vi "Parameter_2nd_part.vi"(6 "Biometry Configuration":T1, 7 "测试？":bool, 8 "Error In":errorcluster caption="错误输入", 9 "A\\B":dbl[](array[numeric]), 10 "Correction Data 2nd":dbl[](array[numeric]), 11 "S":dbl[](array[numeric])) -> (0 "Error Out":errorcluster caption="错误输出", 1 "最值位置":dbl, 2 "开始位置":dbl, 3 "视网膜厚度":dbl)   [LabVIEW 2015, in "Boimetry Processing.lvlib"]
doc: "计算眼后节结果。"
uses:
  Boimetry Processing.lvlib
  Controls/Biometry Configuration.ctl
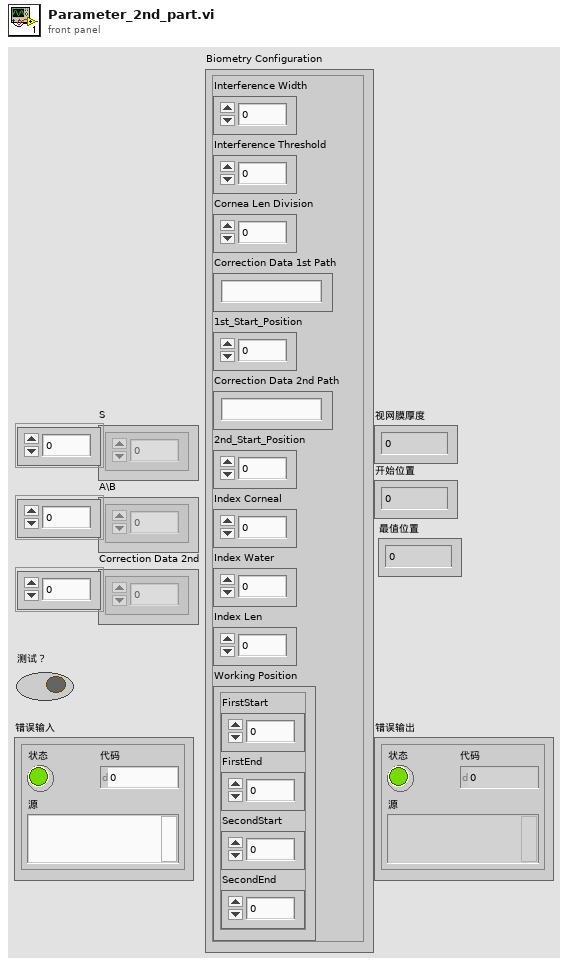
[diagram p1: front panel]
types:
  T1 = typedef "Boimetry Processing.lvlib/Biometry Configuration.ctl" = cluster{"Interference Width":i32, "Interference Threshold":dbl, "Cornea Len Division":i32, "Correction Data 1st Path":string, "1st_Start_Position":dbl, "Correction Data 2nd Path":string, "2nd_Start_Position":dbl, "Index Corneal":dbl, "Index Water":dbl, "Index Len":dbl, "Working Position":cluster{"FirstStart":i32, "FirstEnd":i32, "SecondStart":i32, "SecondEnd":i32}}
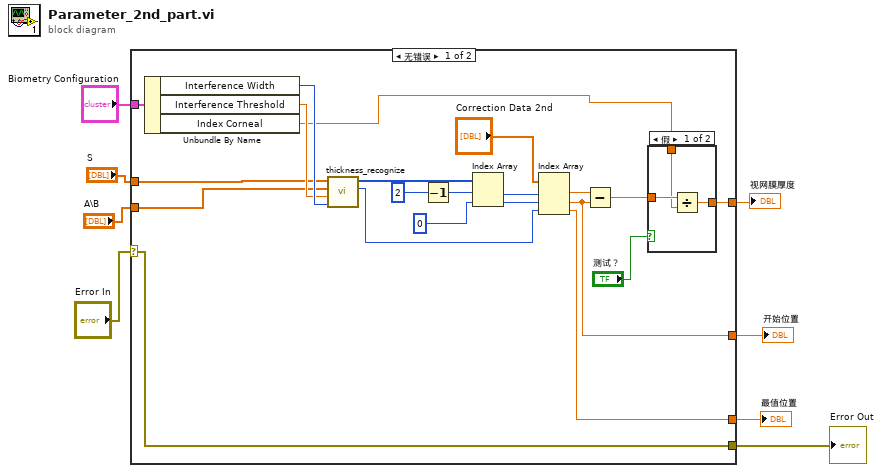
[diagram p0: block diagram]
diagram:
  n1 = case shown="无错误" "Error In" {
    selector: "Error In" -> [w16 w34]
    tunnel: [w21 _] -> w8
    tunnel: [w20 _] -> w7
    tunnel: [w18 _] -> w6
    tunnel: [w16 w34] -> w4
    tunnel: "Biometry Configuration" -> [w14 _]
    tunnel: "S" -> [w10 _]
    tunnel: "A\\B" -> [w9 _]
    frame No Error {
      n2 = Unbundle By Name(w14) -> ("Interference Width"=w13:i32, "Interference Threshold"=w12:dbl, "Index Corneal"=w11:dbl)
      n3 = call "thickness_recognize.vi"("干涉宽度"=w13, "干涉阈值"=w12, "A"=w9, "S"=w10) -> ("MAX_Index"=w19:i32, "INDEX"=w24:i32[])  [unwired: 5 in, 1 out]
      n4 = Decrement(x=2) -> (x-1=w26:i32)
      n5 = Index Array(array=w24, index #1=w26, index #2=0 ("索引")) -> (element #1=w28:i32, element #2=w27:i32)
      n6 = Index Array(array="Correction Data 2nd", index #1=w28, index #2=w27, index #3=w19) -> (element #1=w23:dbl, element #2=w20:dbl, element #3=w18:dbl)
      n7 = Subtract(x=w23, y=w20) -> (x-y=w22:dbl)
      n8 = case shown="假" "测试？" {
        tunnel: w22 -> [w32 w33]
        tunnel: w11 -> [w31 _]
        tunnel: [w30 w33] -> w21
        frame False {
          n9 = Divide(x=w32, y=w31) -> (x/y=w30:dbl)
        }
        frame True {
        }
      }
    }
    frame Error {
    }
  }
  "视网膜厚度" <- w8
  "开始位置" <- w7
  "最值位置" <- w6
  "Error Out" <- w4
